vi "Register Test.vi"(8 "error in (no error)":errorcluster, 10 "VI Call Chain":string[](array[string]), 11 "Assert Factory in":refnum<class "Assert Factory.lvclass">) -> (0 "error out":errorcluster, 3 "Assert Factory out":refnum<class "Assert Factory.lvclass">)   [LabVIEW 2009, in "Caraya.lvlib" / "Assert Factory.lvclass"]
doc: "Registers a Test VI with the Assert Factory"
uses:
  Assert Factory.lvclass
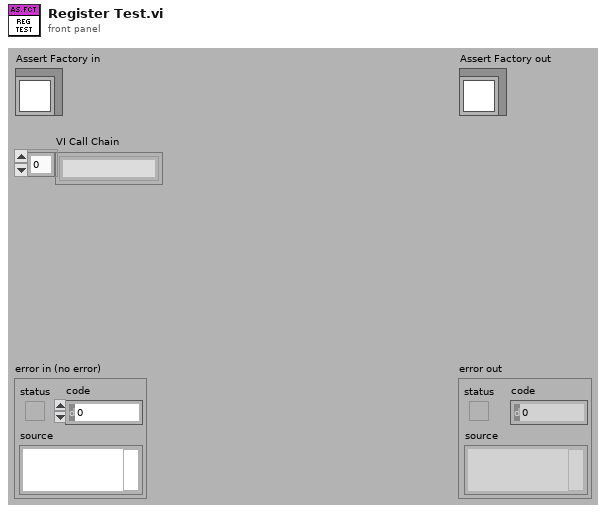
[diagram p1: front panel]
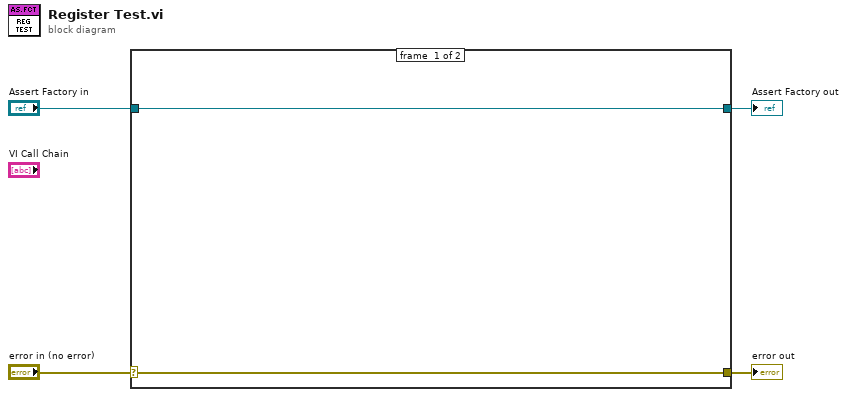
[diagram p0: block diagram]
diagram:
  n1 = case shown="No Error" "error in (no error)" {
    selector: "error in (no error)" -> [w5 w8]
    tunnel: [w5 w8] -> w3
    tunnel: [w6 w7] -> w1
    tunnel: "Assert Factory in" -> [w6 w7]
    frame #0 {
    }
    frame #1 {
    }
  }
  "error out" <- w3
  "Assert Factory out" <- w1
